vi "monodrive_camera.vi"(11 "connection ID":refnum<k5>) -> ()   [LabVIEW 2018]
panel:
  in  "error in (no error)":errorcluster
  out "Follower Camera":picture
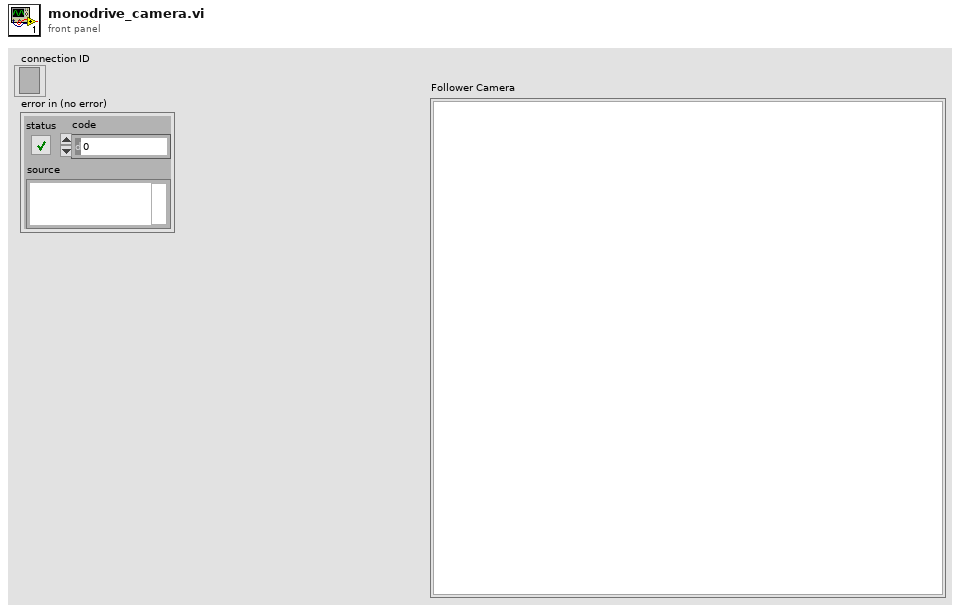
[diagram p1: front panel]
types:
  T1 = typedef "imagedata.ctl" = cluster{"image type":i32, "image depth":i32, "image":u8[], "mask":u8[], "colors":u32[], "Rectangle":cluster{"left":i16, "top":i16, "right":i16, "bottom":i16}}
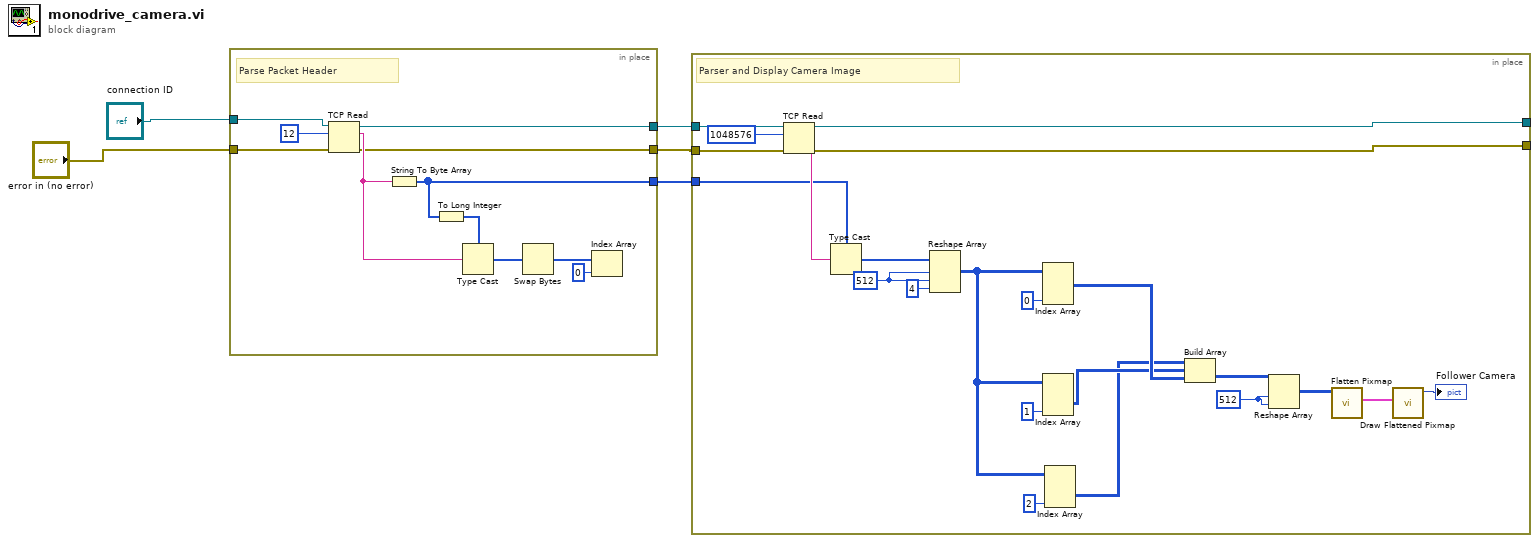
[diagram p0: block diagram]
diagram:
  n1 = in-place "Parse Header" {
    in-place-border: [w13] -> w5
    in-place-border: [w12] -> w4
    in-place-border: [w10] -> w3
    in-place-border: "connection ID" -> [w7]
    in-place-border: "error in (no error)" -> [w6]
    # "Parse Packet Header"
    n2 = TCP Read(connection ID=w7, bytes to read=12, error in (no error)=w6) -> (connection ID out=w13:refnum<k5>, data out=w15:string, error out=w12:errorcluster)  [unwired: 2 in]
    n3 = String To Byte Array(string=w15) -> (unsigned byte array=w10:u8[])
    n4 = To Long Integer(number=w10) -> (32bit integer=w16:i32[])
    n5 = Type Cast(type=w16, x=w15) -> (*(type *) &x=w14:i32[])
    n6 = Swap Bytes(anything=w14) -> (byte swapped=w11:i32[])
    n7 = Index Array(array=w11, index=0) -> ()  [unwired: 1 out]
  }
  n8 = in-place {
    in-place-border: w5 -> [w38]
    in-place-border: w4 -> [w37]
    in-place-border: w3 -> [w35]
    in-place-border: [w28] -> _
    in-place-border: [w27] -> _
    w26 = 512 ("dimension size")
    w34 = 512 ("dimension size")
    # "Parser and Display Camera Image"
    n9 = TCP Read(connection ID=w38, bytes to read=1048576, error in (no error)=w37) -> (connection ID out=w28:refnum<k5>, data out=w36:string, error out=w27:errorcluster)  [unwired: 2 in]
    n10 = Type Cast(type=w35, x=w36) -> (*(type *) &x=w18:u8[])
    n11 = Reshape Array(w18, w34, w34, 4 ("dimension size")) -> (w29:u8[][][])
    n12 = Index Array(array=w29, index (dim 2)=0 ("disabled index (col)")) -> (element=w21:u8[][])  [unwired: 2 in]
    n13 = Index Array(array=w29, index (dim 2)=1 ("index (col)")) -> (element=w20:u8[][])  [unwired: 2 in]
    n14 = Index Array(array=w29, index (dim 2)=2 ("index (col)")) -> (element=w19:u8[][])  [unwired: 2 in]
    n15 = Build Array(w19, w20, w21) -> (w25:u8[][][])
    n16 = Reshape Array(w25, w26, w26) -> (w22:u8[][])
    n17 = call <vilib>:"Flatten Pixmap.vi"("24-bit pixmap"=w22) -> ("image data"=w23:T1)  [unwired: 10 in]
    n18 = call <vilib>:"Draw Flattened Pixmap.vi"("image data"=w23) -> ("new picture"=→"Follower Camera":picture)  [unwired: 8 in]
  }
